vi "Lezeti_Power_Monitor_08.vi"() -> ()   [LabVIEW 2012]
uses:
  <vilib>/Utility/file.llb/Write To Spreadsheet File (DBL).vi
  <instrlib>/RIGOL DS1000 Series/Public/Data/Read (Multiple Waveforms).vi
  <instrlib>/RIGOL DS1000 Series/RIGOL DS1000 Series.lvlib
panel:
  in  "Attenunation2":dbl
  in  "Attenuation 1":dbl
  in  "Path":path
  in  "Coupling 2":dbl
  in  "Coupling 1":dbl
  in  "Channel 2":dbl
  out "Waveform Graph":waveform(dbl)[](graph)
  in  "Iteration Time":dbl
  in  "Timeout":dbl
  in  "Channel":dbl
  in  "stop":bool
  in  "VISA resource name":refnum<visa-resource-name>
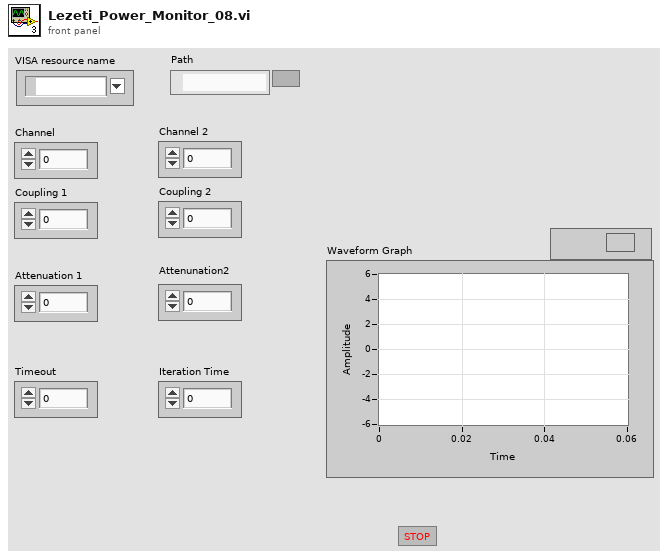
[diagram p1: front panel]
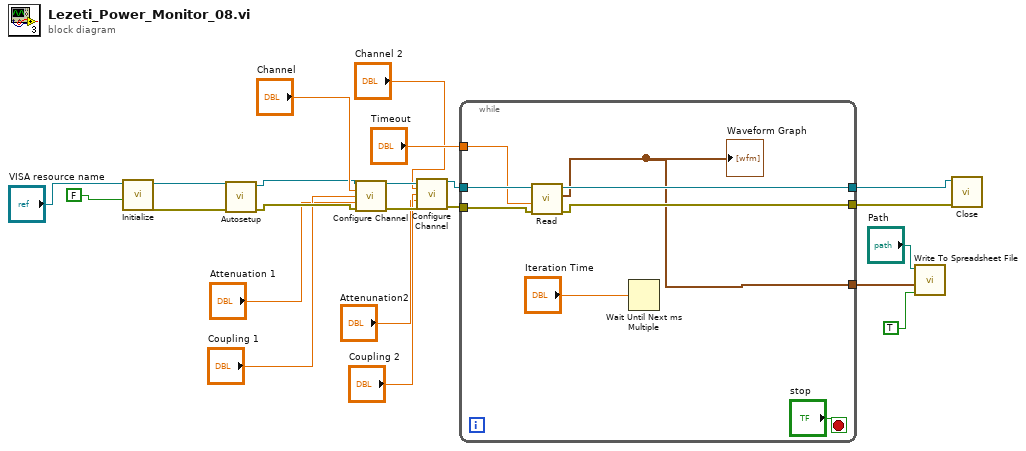
[diagram p0: block diagram]
diagram:
  n1 = call <instrlib>:"Initialize.vi"("Reset (True)"=FALSE, "VISA resource name"="VISA resource name") -> ("error out"=w9:errorcluster, "VISA resource name out"=w10:refnum<visa-resource-name>)  [unwired: 8 in]
  n2 = call <instrlib>:"Autosetup.vi"("error in (no error)"=w9, "VISA resource name"=w10) -> ("error out"=w7:errorcluster, "VISA resource name out"=w8:refnum<visa-resource-name>)  [unwired: 8 in]
  n3 = call <instrlib>:"Configure Channel.vi"("VISA resource name"=w8, "Channel (1: Channel 1)"="Channel", "Vertical Coupling (0: DC)"="Coupling 1", "Probe Attenuation (1.0)"="Attenuation 1", "error in (no error)"=w7) -> ("VISA resource name out"=w17:refnum<visa-resource-name>, "error out"=w16:errorcluster)  [unwired: 9 in]
  n4 = call <instrlib>:"Configure Channel.vi"("VISA resource name"=w17, "Channel (1: Channel 1)"="Channel 2", "Vertical Coupling (0: DC)"="Coupling 2", "Probe Attenuation (1.0)"="Attenunation2", "error in (no error)"=w16) -> ("VISA resource name out"=w15:refnum<visa-resource-name>, "error out"=w14:errorcluster)  [unwired: 9 in]
  n5 = while {
    tunnel: w14 -> [w29]
    tunnel: w15 -> [w28]
    tunnel: [w27] -> w20
    tunnel: [w26] -> w19
    tunnel: "Timeout" -> [w25]
    tunnel: [w23] -> w11
    stop <- "stop" stop-if-true
    n6 = call-poly <instrlib>:"Read.vi"("error in (no error)"=w29, "Timeout (10000 ms)"=w25, "VISA resource name"=w28) -> ("error out"=w26:errorcluster, "Waveform Data"=w23:waveform(dbl)[], "VISA resource name out"=w27:refnum<visa-resource-name>)  [unwired: 6 in]
    "Waveform Graph" <- w23
    n7 = Wait Until Next ms Multiple(millisecond multiple="Iteration Time") -> ()  [unwired: 1 out]
  }
  n8 = call-poly <vilib>:"Write To Spreadsheet File.vi"("append to file? (new file:F)"=TRUE, "1D data"=w11, "file path (dialog if empty)"="Path") -> ()  [unwired: 5 in, 1 out]
  n9 = call <instrlib>:"Close.vi"("error in (no error)"=w19, "VISA resource name"=w20) -> ()  [unwired: 9 in, 1 out]
